vi "pp_stiimList_createPseudoGellerman.vi"(8 "error in (no error)":errorcluster, 10 "Total Trials":i32=60 min=2 step=2, 11 "Trial Types":T1(array[cluster]) {"Stim P2" min=0.0; "Trial Weight" step=1; "Stim P1" min=0.0; "Stim Dur (s)" min=0.0; "Trial Code" min=1 step=1}) -> (0 "error out":errorcluster, 3 "Session List (Cannot Edit)":i32[](array[numeric]))   [LabVIEW 2013]
uses:
  labolabo/random/impl/RandomizeArray_I.vi
  labolabo/array/impl/NullArray_I.vi
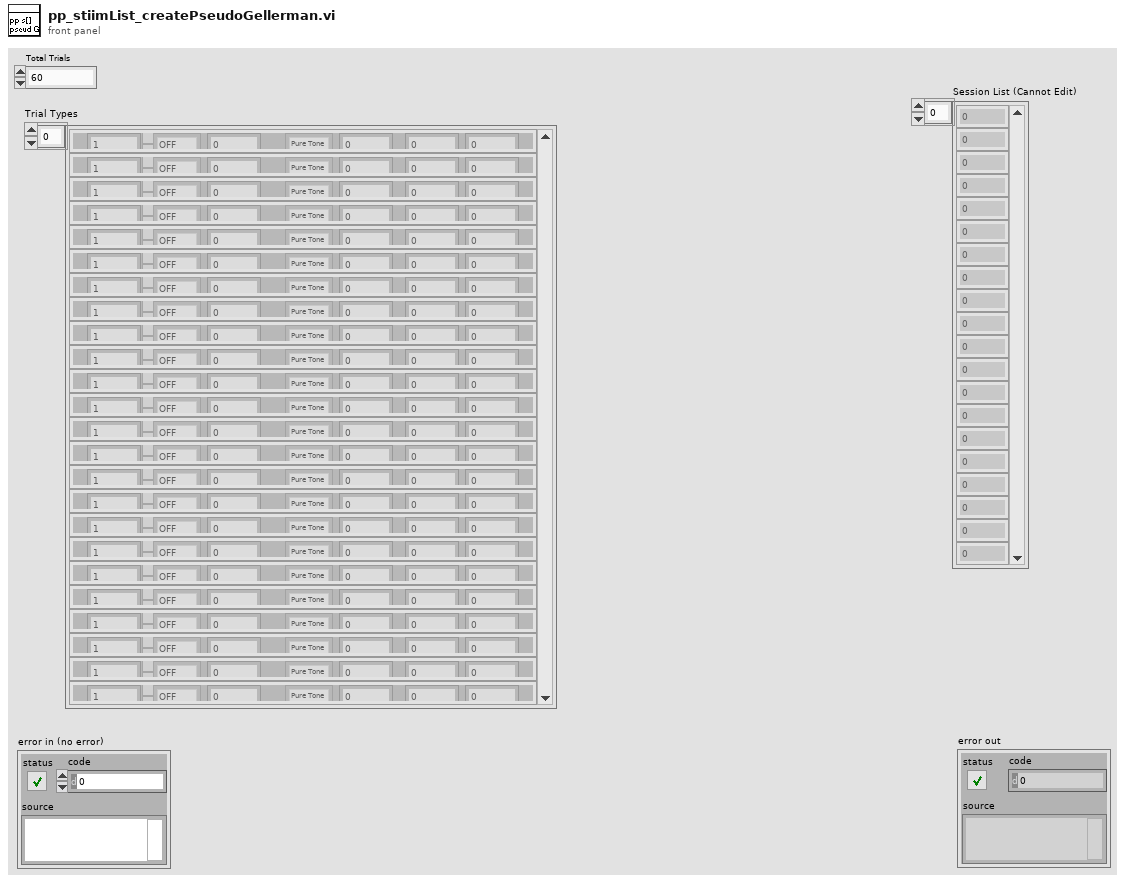
[diagram p1: front panel]
types:
  T1 = cluster{"Trial Code":u16, "Trial Type":enum16{"OFF", "GO", "NOGO", "TEST"}, "Trial Weight":u32, "Stim Type":enum16{"Pure Tone", "FM Sweep"}, "Stim Dur (s)":dbl, "Stim P1":dbl, "Stim P2":dbl}[]
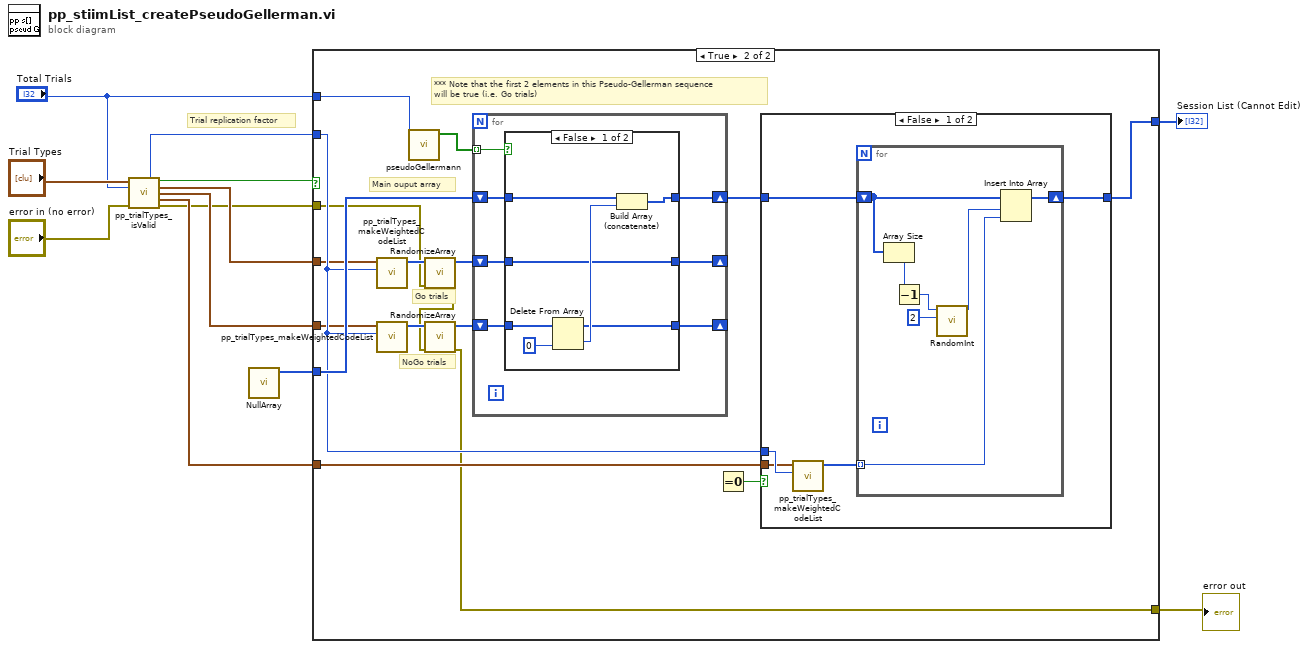
[diagram p0: block diagram]
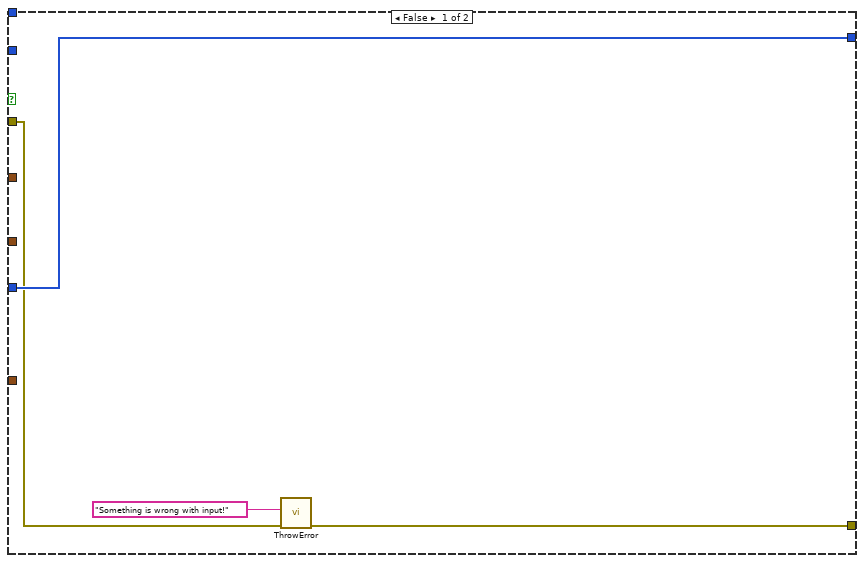
[diagram p2: hidden frame]
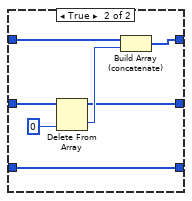
[diagram p4: hidden frame]
diagram:
  # "Trial replication factor"
  n1 = call "pp_trialTypes_isValid.vi"("Trial Types"="Trial Types", "Total Trials"="Total Trials", "error in (no error)"="error in (no error)") -> ("Trial Replication Factor"=w7:i32, "Paradigm Valid?"=w5:bool, "GO Trials"=w4:T1, "NOGO Trials"=w3:T1, "TEST Trials"=w2:T1, "error out"=w1:errorcluster)  [unwired: 7 in]
  n2 = call-poly "NullArray.vi"() -> ("Null Array"=w12:i32[])  [unwired: 11 in]
  n3 = case shown="True" w5 {
    tunnel: w7 -> [_ w23]
    tunnel: "Total Trials" -> [_ w33]
    tunnel: w12 -> [w16 w27]
    tunnel: [w16 w24] -> w11
    tunnel: [w14 w17] -> w10
    tunnel: w4 -> [_ w22]
    tunnel: w3 -> [_ w21]
    tunnel: w2 -> [_ w20]
    tunnel: w1 -> [w13 w19]
    frame False {
      n4 = call "ThrowError.vi"("error in (no error)"=w13, "Error Message"="Something is wrong with input!" ("error message (\"\")")) -> ("error out"=w14:errorcluster)  [unwired: 8 in, 1 out]
    }
    frame True {
      # "*** Note that the first 2 elements in this Pseudo-Gellerman sequence\nwill be true (i.e. Go trials)"
      # "NoGo trials"
      # "Go trials"
      # "Main ouput array"
      n5 = call "pp_trialTypes_makeWeightedCodeList.vi"("Trial Replication Factor"=w23, "Trial Types"=w22) -> ("Weighted Code List"=w30:i32[])  [unwired: 9 in]
      n6 = call "pp_trialTypes_makeWeightedCodeList.vi"("Trial Replication Factor"=w23, "Trial Types"=w21) -> ("Weighted Code List"=w29:i32[])  [unwired: 9 in]
      n7 = call "pseudoGellermann.vi"("N"=w33) -> ("Array"=w32:bool[])  [unwired: 10 in]
      n8 = call-poly "RandomizeArray.vi"("error in (no error)"=w19, "Array In"=w30) -> ("error out"=w18:errorcluster, "Array Out"=w31:i32[])  [unwired: 8 in]
      n9 = call-poly "RandomizeArray.vi"("error in (no error)"=w18, "Array In"=w29) -> ("error out"=w17:errorcluster, "Array Out"=w28:i32[])  [unwired: 8 in]
      n10 = for {
        tunnel: w32 -> [w53] mode=indexing
        shift-right: [w48] -> _
        shift-left: w31 -> [w49]
        shift-right: [w50] -> _
        shift-left: w28 -> [w51]
        shift-right: [w47] -> w25
        shift-left: w27 -> [w52]
        n11 = case shown="False" w53 {
          tunnel: [w59 w66] -> w47
          tunnel: w52 -> [w58 w65]
          tunnel: w51 -> [w56 w64]
          tunnel: [w55 w64] -> w50
          tunnel: w49 -> [w54 w63]
          tunnel: [w54 w61] -> w48
          frame False {
            n12 = Delete From Array(array=w56, index=0 ("index (row)")) -> (deleted portion=w57:i32, array with subset deleted=w55:i32[])  [unwired: 1 in]
            n13 = Build Array (concatenate)(w58, w57) -> (w59:i32[])
          }
          frame True {
            n14 = Delete From Array(array=w63, index=0 ("index (row)")) -> (deleted portion=w62:i32, array with subset deleted=w61:i32[])  [unwired: 1 in]
            n15 = Build Array (concatenate)(w65, w62) -> (w66:i32[])
          }
        }
      }
      n16 = Equal To 0?() -> (x = 0?=w26:bool)  [unwired: 1 in]
      n17 = case shown="False" w26 {
        tunnel: w25 -> [w36 w46]
        tunnel: [w35 w46] -> w24
        tunnel: w23 -> [w38 _]
        tunnel: w20 -> [w34 _]
        frame False {
          n18 = call "pp_trialTypes_makeWeightedCodeList.vi"("Trial Replication Factor"=w38, "Trial Types"=w34) -> ("Weighted Code List"=w37:i32[])  [unwired: 9 in]
          n19 = for {
            tunnel: w37 -> [w40] mode=indexing
            shift-right: [w41] -> w35
            shift-left: w36 -> [w42]
            n20 = Array Size(array=w42) -> (size(s)=w43:i32)
            n21 = Decrement(x=w43) -> (x-1=w44:i32)
            n22 = call "RandomInt.vi"("Min"=2, "Max"=w44) -> ("Random"=w39:i32)  [unwired: 9 in]
            n23 = Insert Into Array(array=w42, index=w39, new element=w40) -> (w41:i32[])
          }
        }
        frame True {
        }
      }
    }
  }
  "error out" <- w10
  "Session List (Cannot Edit)" <- w11
